vi "IIR Filter by N Specs for N Chan.vi"(4 "optional IIR filter specifications":T3(array[cluster]) {"PB Gain" format="%0.2f"; "SB Gain" format="%0.2f"; "Lower SB" format="%0.2p"; "Upper SB" format="%0.2f"; "Lower PB" format="%0.2p"; "Upper PB" format="%0.2f"}, 6 "IIR filter specifications":T4(array[cluster]) {"PB Ripple" format="%0.2f"; "SB Attenuation" format="%0.2f"; "Lower Fc" format="%0.2p"; "Upper Fc" format="%0.2p"}, 7 "reset filters":bool, 8 "error in (no error)":errorcluster, 10 "filter structure option":T1=10 items=["IIR 2nd Order"=0, "IIR 4th Order"=1, "Auto Select"=10], 11 "signal(s) in":waveform(dbl)[](array[waveform])) -> (0 "error out":errorcluster, 2 "filter information":T2(array[cluster]) {"phase H(w)"."df" format="%0.2f"; "phase H(w)"."f0" format="%0.2f"; "phase H(w)"."Phase H(w)" format="%0.2f"; "magnitude H(w)"."df" format="%0.2f"; "magnitude H(w)"."f0" format="%0.2f"; "magnitude H(w)"."Mag H(w)" format="%0.2f"}, 3 "signal(s) out":waveform(dbl)[](array[waveform]))   [LabVIEW 2020, in "NI_MAPro.lvlib"]
doc: "Filters signals in either single or multiple waveforms. If you are filtering multiple waveforms, the VI maintains separate filter states for each waveform. The data types you wire to the <B>signal in</B> and <B>IIR filter specifications</B> inputs determine the polymorphic instance to use."
uses:
  NI_MAPro.lvlib
  Filter Structure Type.ctl
  NI_MABase.lvlib
  NI_AALBase.lvlib
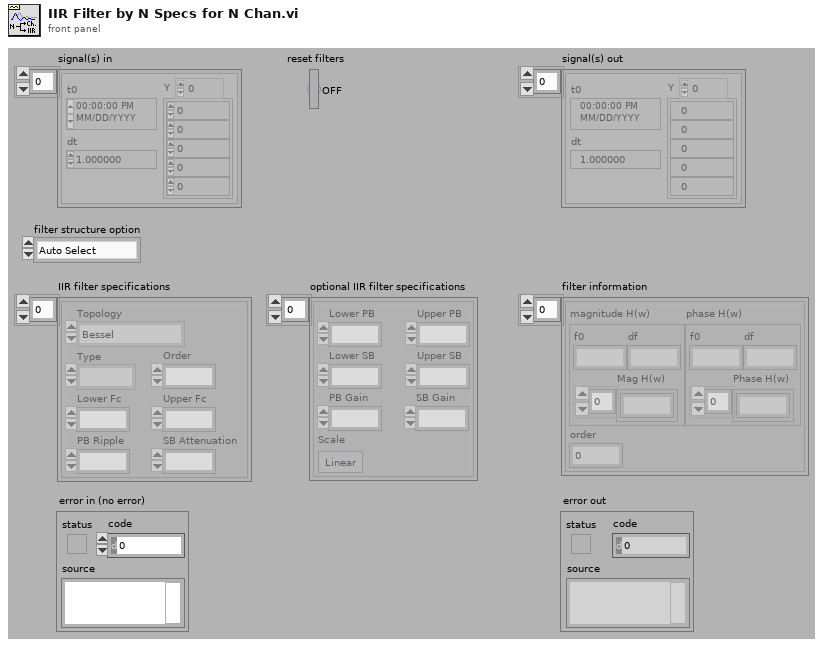
[diagram p1: front panel]
types:
  T1 = typedef "NI_AALBase.lvlib/Filter Structure Type.ctl" = u16
  T2 = cluster{"magnitude H(w)":cluster{"f0":dbl, "df":dbl, "Mag H(w)":dbl[]}, "phase H(w)":cluster{"f0":dbl, "df":dbl, "Phase H(w)":dbl[]}, "order":i32}[]
  T3 = cluster{"Lower PB":dbl, "Upper PB":dbl, "Lower SB":dbl, "Upper SB":dbl, "PB Gain":dbl, "SB Gain":dbl, "Scale":bool}[]
  T4 = cluster{"Topology":enum16{"Off", "Butterworth", "Chebyshev", "Inverse Chebyshev", "Elliptic", "Bessel"}, "Type":enum16{"Lowpass", "Highpass", "Bandpass", "Bandstop"}, "Order":i32, "Lower Fc":dbl, "Upper Fc":dbl, "PB Ripple":dbl, "SB Attenuation":dbl}[]
  T5 = cluster{"filter structure":enum32{"IIR 2nd Order", "IIR 4th Order"}, "Reverse Coefficients":dbl[], "Forward Coefficients":dbl[]}[]
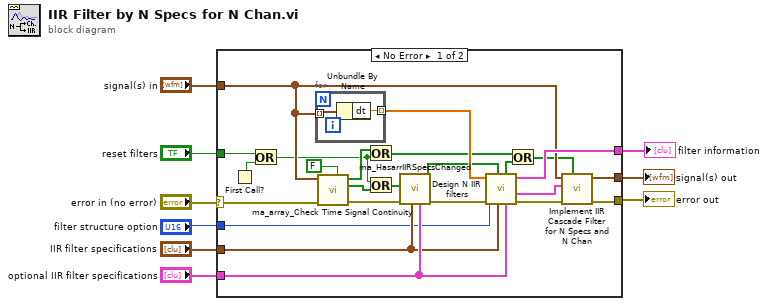
[diagram p0: block diagram]
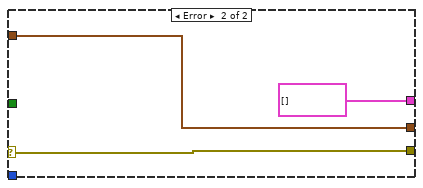
[diagram p2: hidden frame]
diagram:
  n1 = case shown="No Error" "error in (no error)" {
    selector: "error in (no error)" -> [w27 w37]
    tunnel: "signal(s) in" -> [w26 w38]
    tunnel: "IIR filter specifications" -> [w20 _]
    tunnel: [w33 w37] -> w8
    tunnel: [w32 w38] -> w7
    tunnel: "optional IIR filter specifications" -> [w21 _]
    tunnel: [w28 T2 [] ("arrFilterInfo")] -> w3
    tunnel: "reset filters" -> [w12 _]
    tunnel: "filter structure option" -> [w10 _]
    frame No Error {
      n2 = First Call?() -> (First Call?: T/F=w13:bool)
      n3 = Or(x=w12, y=w13) -> (x .or. y?=w11:bool)
      n4 = for {
        tunnel: w26 -> [w34] mode=indexing
        tunnel: [w35] -> w29 mode=indexing
        n5 = Unbundle By Name(w34) -> ("dt"=w35:dbl)
      }
      n6 = call "ma_array_Check Time Signal Continuity.vi"("Ignore input time stamp"=FALSE, "error in (no error)"=w27, "waveforms"=w26) -> ("error out"=w22:errorcluster, "dt changed"=w17:bool[], "t0 changed"=w16:bool[])  [unwired: 5 in, 1 out]
      n7 = Or(x=w16, y=w11) -> (x .or. y?=w15:bool[])
      n8 = Or(x=w11, y=w17) -> (x .or. y?=w18:bool[])
      n9 = call "ma_HasarrIIRSpecsChanged.vi"("optional IIR filter specifications"=w21, "IIR filter specs"=w20, "error in (no error)"=w22, "redesign filter"=w18) -> ("error out"=w23:errorcluster, "valsDifferent?"=w19:bool[])  [unwired: 6 in]
      n10 = call "Design N IIR filters.vi"("arrOptionalFilterSpecs"=w21, "arrFilterSpecs"=w20, "redesign filters"=w19, "error in"=w23, "filter structure option"=w10, "arrdt"=w29) -> ("error out"=w30:errorcluster, "arrIIRFilterCluster"=w31:T5, "arrFilterInfo"=w28:T2, "reset filter states"=w25:bool[])  [unwired: 2 in]
      n11 = Or(x=w15, y=w25) -> (x .or. y?=w24:bool[])
      n12 = call "Implement IIR Cascade Filter for N Specs and N Chan.vi"("reset filter states"=w24, "error in (no error)"=w30, "arrIIRFIlterCluster"=w31, "arrWaveforms"=w26) -> ("error out"=w33:errorcluster, "arrFilteredWaveforms"=w32:waveform(dbl)[])  [unwired: 6 in]
    }
    frame Error {
    }
  }
  "error out" <- w8
  "signal(s) out" <- w7
  "filter information" <- w3
